vi "Init SMU.vi"(6 "Init/Config":bool, 8 "error in (no error)":errorcluster, 10 "Channel Name":string="0,1", 11 "IVI Refnum in":refnum<k15>) -> (0 "error out":errorcluster, 3 "IVI Refnum out":refnum<k15>)   [LabVIEW 2018]
uses:
  <instrlib>/niDCPower/nidcpower.llb/niDCPower Source Mode.ctl
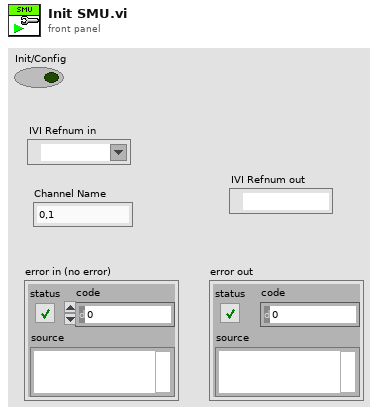
[diagram p1: front panel]
types:
  T1 = typedef "niDCPower Source Mode.ctl" = i32
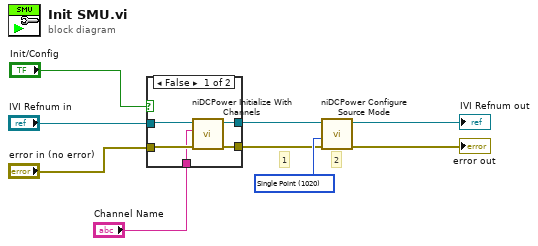
[diagram p0: block diagram]
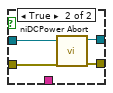
[diagram p2: hidden frame]
diagram:
  w5 = T1 1020 items=["Single Point"=1020, "Sequence"=1021] ("source mode")
  # "1"
  # "2"
  n1 = case shown="False" "Init/Config" {
    tunnel: "error in (no error)" -> [w13 w18]
    tunnel: "IVI Refnum in" -> [w11 w17]
    tunnel: [w12 w16] -> w1
    tunnel: [w14 w15] -> w2
    tunnel: "Channel Name" -> [w10 _]
    frame False {
      n2 = call <instrlib>:"niDCPower Initialize With Channels.vi"("error in (no error)"=w13, "channels"=w10, "resource name"=w11) -> ("error out"=w14:errorcluster, "instrument handle out"=w12:refnum<k15>)  [unwired: 7 in]
    }
    frame True {
      n3 = call <instrlib>:"niDCPower Abort.vi"("error in (no error)"=w18, "instrument handle"=w17) -> ("error out"=w15:errorcluster, "instrument handle out"=w16:refnum<k15>)  [unwired: 8 in]
    }
  }
  n4 = call <instrlib>:"niDCPower Configure Source Mode.vi"("error in (no error)"=w2, "source mode"=w5, "instrument handle"=w1) -> ("error out"=→"error out":errorcluster, "instrument handle out"=→"IVI Refnum out":refnum<k15>)  [unwired: 7 out]
